vi "sigmoid.vi"(1 "x":dbl[][](array[numeric])) -> (0 "y":T1)   [LabVIEW 2020]
uses:
  <vilib>/Analysis/Matrix/Datatypes/RealMatrix.ctl
  <vilib>/Analysis/Matrix/Numeric/Conversions/Array To Matrix - RA.vi
  <vilib>/Analysis/Matrix/NI_Matrix.lvlib
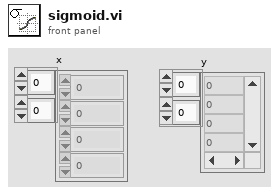
[diagram p1: front panel]
types:
  T1 = typedef "NI_Matrix.lvlib/RealMatrix.ctl" = dbl[][]
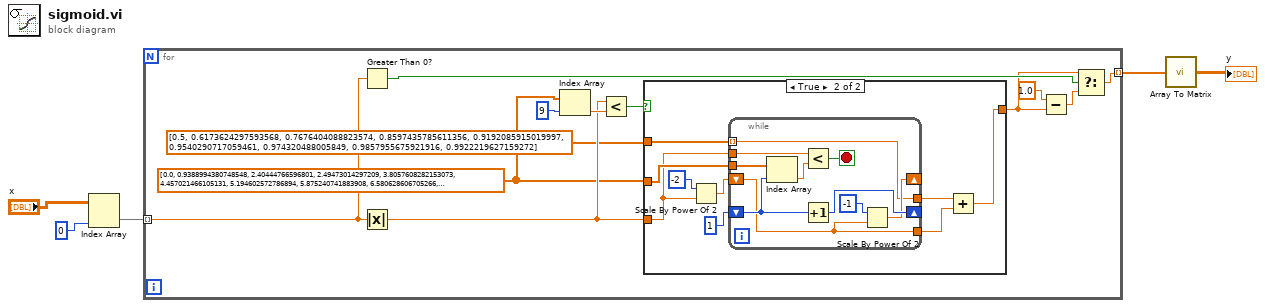
[diagram p0: block diagram]
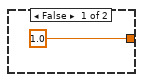
[diagram p2: hidden frame]
diagram:
  n1 = Index Array(array="x", index (col)=0) -> (element=w4:dbl[])  [unwired: 1 in]
  n2 = for {
    tunnel: w4 -> [w13] mode=indexing
    tunnel: [w8] -> w2 mode=indexing
    w7 = dbl[] [0.0, 0.9388994380748548, 2.40444766596801, 2.49473014297209, 3.8057608282153073, 4.457021466105131, 5.194602572786894, 5.875240741883908, 6.580628606705266, 7.9647101788905275]
    n3 = Greater Than 0?(x=w13) -> (x > 0?=w12:bool)
    n4 = Absolute Value(x=w13) -> (abs(x)=w14:dbl)
    n5 = Index Array(array=w7, index=9) -> (element=w16:dbl)
    n6 = Less?(x=w14, y=w16) -> (x < y?=w17:bool)
    n7 = case shown="True" w17 {
      tunnel: w14 -> [_ w20]
      tunnel: [1.0 w26] -> w10
      tunnel: w7 -> [_ w25]
      tunnel: dbl[] [0.5, 0.6173624297593568, 0.7676404088823574, 0.8597435785611356, 0.9192085915019997, 0.9540290717059461, 0.974320488005849, 0.9857955675921916, 0.9922219627159272] -> [_ w24]
      frame False {
      }
      frame True {
        n8 = Scale By Power Of 2(n=-2, x=w20) -> (x*2^n=w19:dbl)
        n9 = while {
          tunnel: w20 -> [w37]
          shift-right: [w35] -> _
          shift-left: 1 -> [w33]
          shift-right: [w32] -> _
          shift-left: w19 -> [w30]
          tunnel: [w30] -> w23
          tunnel: w25 -> [w29]
          tunnel: [w28] -> w22
          tunnel: w24 -> [w28] mode=indexing
          stop <- w36 stop-if-true
          n10 = Index Array(array=w29, index=w33) -> (element=w34:dbl)
          n11 = Less?(x=w37, y=w34) -> (x < y?=w36:bool)
          n12 = Increment(x=w33) -> (x+1=w35:i32)
          n13 = Scale By Power Of 2(n=-1, x=w30) -> (x*2^n=w32:dbl)
        }
        n14 = Add(x=w22, y=w23) -> (x+y=w26:dbl)
      }
    }
    n15 = Subtract(x=1.0, y=w10) -> (x-y=w9:dbl)
    n16 = Select(t=w10, s=w12, f=w9) -> (s? t:f=w8:dbl)
  }
  n17 = call-poly <vilib>:"Array To Matrix.vi"("Real 1D Array"=w2) -> ("Real Matrix (Column Vector)"=→"y":T1)
